vi "PID tester gyro.vi"   [LabVIEW 2016]
types:
  T1 = typedef "LVHSConnector.ctl" = refnum<class "BrickReference.lvclass">
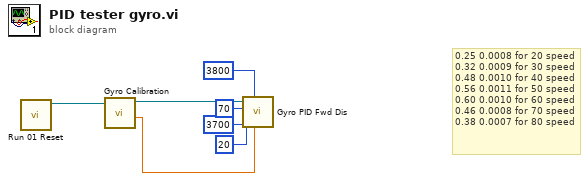
[diagram p0: block diagram]
diagram:
  # "0.25 0.0008 for 20 speed\n0.32 0.0009 for 30 speed\n0.48 0.0010 for 40 speed\n0.56 0.0011 for 50 speed\n0.60 0.0010 for 60 speed\n0.46 0.0008 for 70 speed\n0.38 0.0007 for 80 speed"
  n1 = call "Run 01 Reset.vi"() -> ("NXT/EV3 out"=w2:T1)  [unwired: 11 in]
  n2 = call "Gyro Calibration.vi"("NXT/EV3"=w2) -> ("Degrees"=w5:sgl, "NXT/EV3"=w6:T1)  [unwired: 6 in, 1 out]
  n3 = call "Gyro PID Fwd Dis.vi"("Target angle"=w5, "Threshold to stop"=3800, "Threshold to slow"=3700, "Min. speed"=20, "Max. speed"=70, "EV3 in"=w6) -> ()  [unwired: 5 in, 1 out]
